vi "SA5G_runAlignment.vi"(8 "error in":errorcluster, 11 "VISA in":refnum<visa-resource-name>) -> (0 "error out":errorcluster, 2 "SA_Resp":string, 3 "VISA out":refnum<visa-resource-name>)   [LabVIEW 2020, in "Keysight.lvlib"]
uses:
  Keysight.lvlib
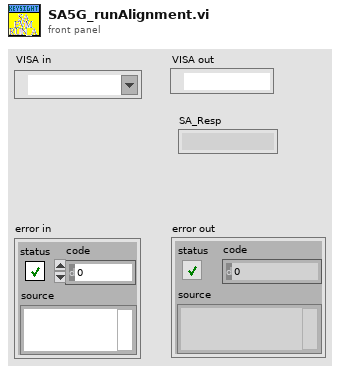
[diagram p1: front panel]
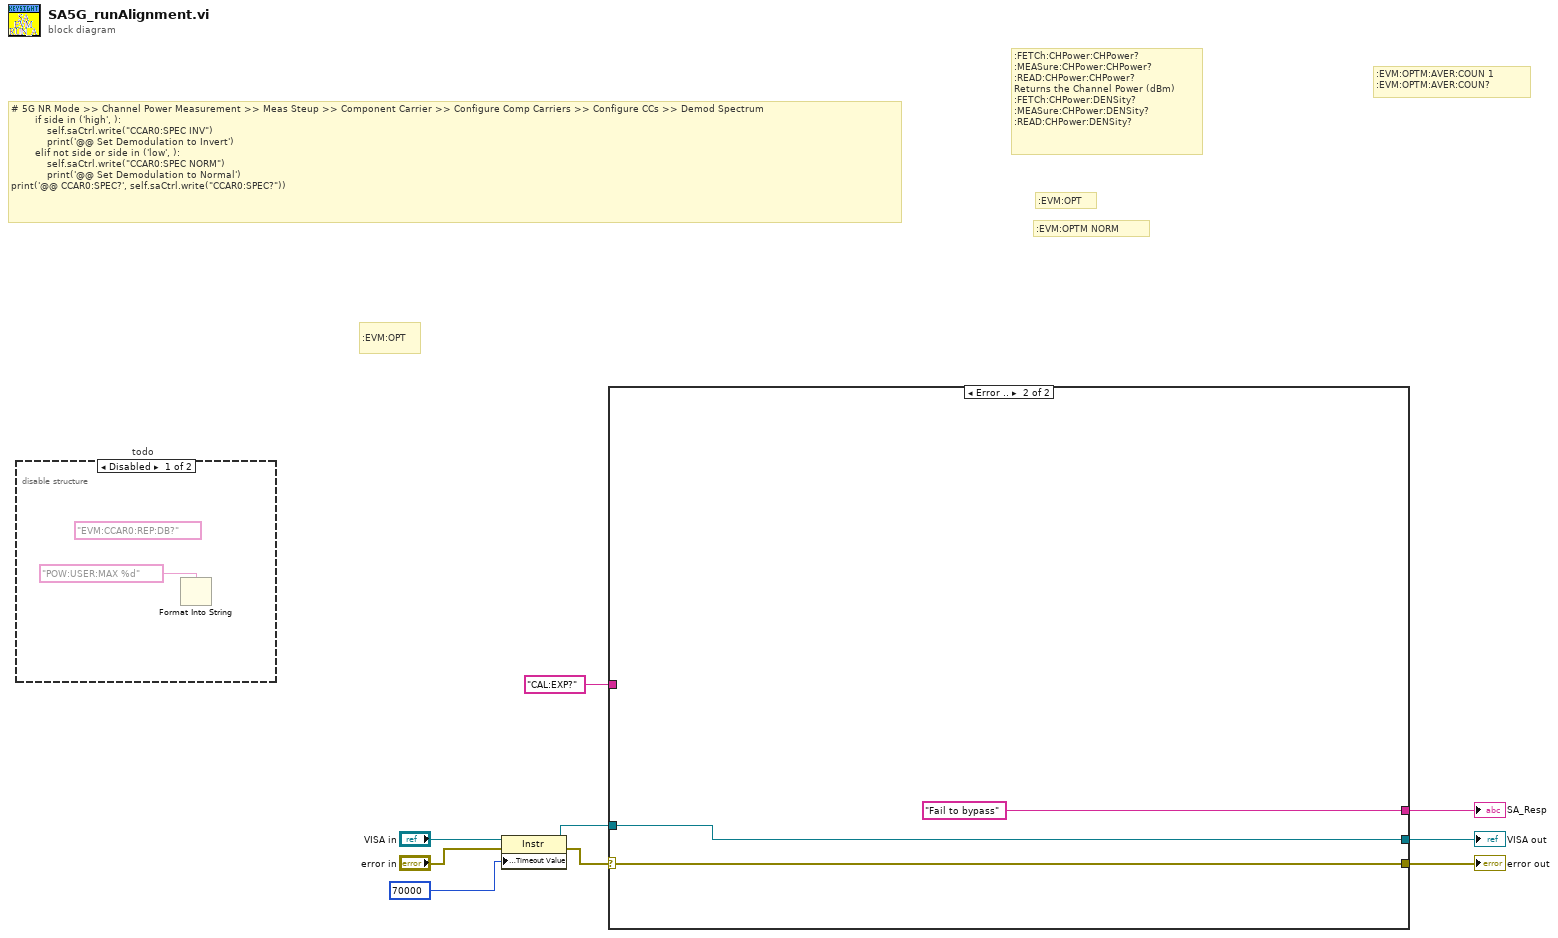
[diagram p0: block diagram]
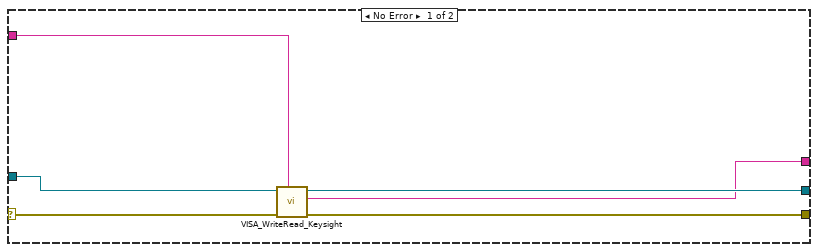
[diagram p3: hidden frame]
diagram:
  # ":EVM:OPTM NORM"
  # ":EVM:OPTM:AVER:COUN 1\n:EVM:OPTM:AVER:COUN?"
  # ":EVM:OPT"
  # ":FETCh:CHPower:CHPower?\n:MEASure:CHPower:CHPower?\n:READ:CHPower:CHPower?\nReturns the Channel Power (dBm)\n:FETCh:CHPower:DENSity?\n:MEASure:CHPower:DENSity?\n:READ:CHPower:DENSity?"
  # ":EVM:OPT"
  # "# 5G NR Mode >> Channel Power Measurement >> Meas Steup >> Component Carrier >> Configure Comp Carriers >> Configure CCs >> Demod Spectrum\n        if side in ('high', ):\n            self.saCtrl.write(\"CCAR0:SPEC INV\")\n            print('@@ Set Demodulation to Invert')\n        elif not side or side in ('low', ):\n            self.saCtrl.write(\"CCAR0:SPEC NORM\")\n            print('@@ Set Demodulation to Normal')\nprint('@@ CCAR0:SPEC?', self.saCtrl.write(\"CCAR0:SPEC?\"))"
  n1 = disable-structure "todo" shown="Disabled" {
    frame Disabled {
      (unwired) "EVM:CCAR0:REP:DB?" ("write buffer")
      n2 = Format Into String(format string="POW:USER:MAX %d") -> ()  [unwired: 3 in, 2 out]
    }
    frame Enabled {
    }
  }
  n3 = property on="Property Node" class="Instr"(reference="VISA in", error in="error in", "General Settings:Timeout Value"=u32 70000) -> (reference out=w1:refnum<visa-resource-name>, error out=w2:errorcluster)
  n4 = case shown="Error .." w2 {
    selector: w2 -> [w12 w19]
    tunnel: [w16 w19] -> w7
    tunnel: [w15 w17] -> w8
    tunnel: [w14 "Fail to bypass" ("Response")] -> w9
    tunnel: "CAL:EXP?" ("write buffer") -> [w13 _]
    tunnel: w1 -> [w11 w17]
    frame No Error {
      n5 = call "VISA_WriteRead_Keysight.vi"("VISA_CMD"=w13, "error in"=w12, "VISA in"=w11) -> ("error out"=w16:errorcluster, "Response"=w14:string, "VISA out"=w15:refnum<visa-resource-name>)  [unwired: 6 in]
    }
    frame Error {
    }
  }
  "SA_Resp" <- w9
  "VISA out" <- w8
  "error out" <- w7
